vi "Config Spark Max SLOT SmartMotion HW Get Set.vi"(4 "PIDF Slot (0)":i32, 6 "Get(f) Set(t)":bool, 7 "SparkMax Slot SM":T1={"Max Velocity"=0.0, "Max Acceleration"=1.0, "Allowed CL Error"=0.0, "Min Velocity Output"=0.0}, 8 "Error":errorcluster, 11 "Drive Refs":T2) -> (0 "Error Out":errorcluster, 3 "Drive Refs Out":T2, 5 "SparkMax Slot SM Out":T1={"Max Velocity"=0.0, "Max Acceleration"=1.0, "Allowed CL Error"=0.0, "Min Velocity Output"=0.0})   [LabVIEW 2023, in "Swerve AM_ACT.lvlib"]
uses:
  Swerve AM_ACT.lvlib
  <vilib>/Rock Robotics/WPI/MotorControl/WPI_MotorControlDeviceRef.ctl
  <vilib>/Rock Robotics/WPI/MotorControl/WPI_MotorControlType.ctl
  <vilib>/Rock Robotics/SystemInterfaces/DIO/FPGA_DIOPWMChannel.ctl
  <vilib>/Rock Robotics/WPI/PWM/WPI_PWMDeadband.ctl
  <vilib>/Rock Robotics/SystemInterfaces/DIO/FPGA_DIOChannel.ctl
  Shared Code/TypeDefs/Cluster_SparkMax Smart Motion Parameters.ctl
  Shared Code/TypeDefs/Cluster_SRX SLOT PID Config.ctl
  Shared Code/TypeDefs/Cluster_PID Gains.ctl
  <vilib>/Utility/error.llb/Trim Whitespace One-Sided.vi
  <vilib>/Utility/Data Type/NI_Data Type.lvlib
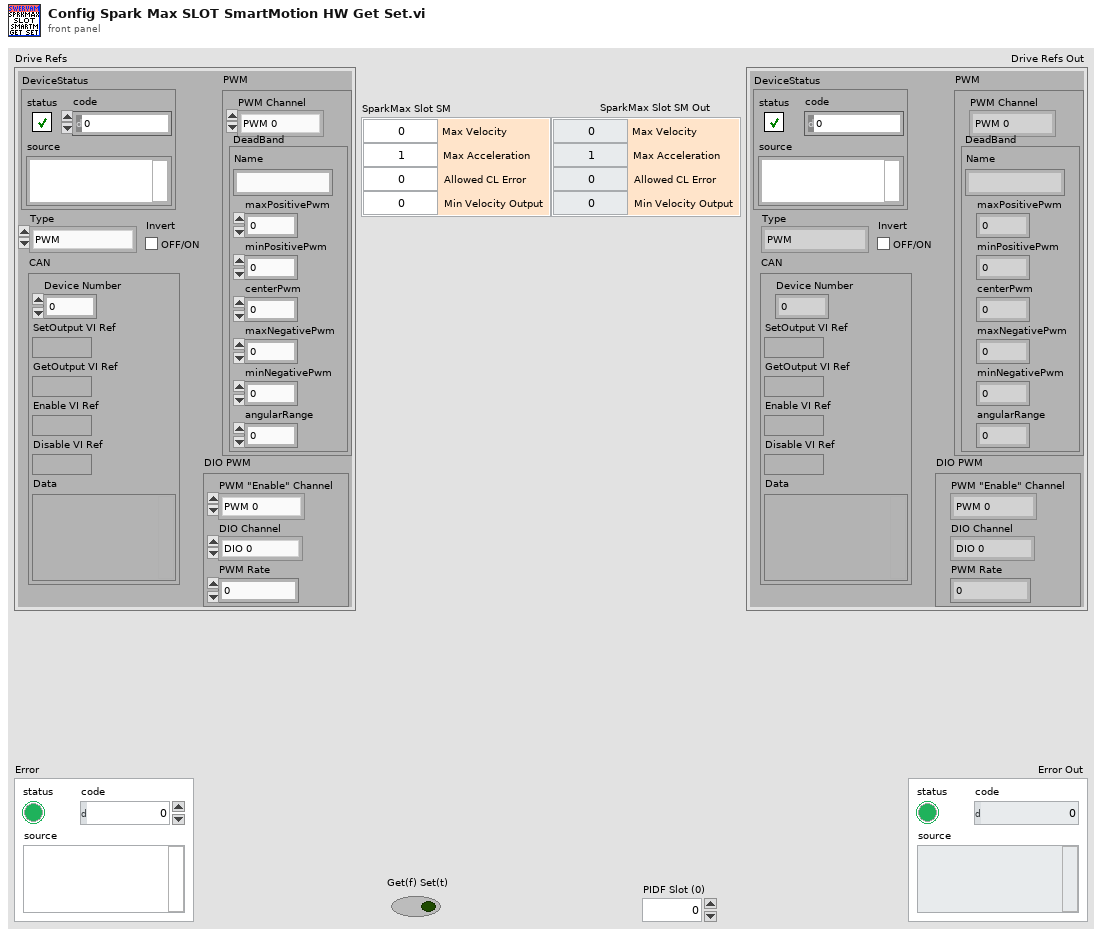
[diagram p1: front panel]
types:
  T1 = typedef "Cluster_SparkMax Smart Motion Parameters.ctl" = cluster{"Max Velocity":dbl, "Max Acceleration":dbl, "Allowed CL Error":dbl, "Min Velocity Output":dbl}
  T2 = typedef "WPI_MotorControlDeviceRef.ctl" = cluster{"DeviceStatus":errorcluster, "Type":T3, "PWM":cluster{"PWM Channel":T4, "DeadBand":T5}, "CAN":cluster{"Device Number":u8, "SetOutput VI Ref":variant, "GetOutput VI Ref":variant, "Enable VI Ref":variant, "Disable VI Ref":variant, "Data":variant}, "Invert":bool, "DIO PWM":cluster{"PWM \"Enable\" Channel":T4, "DIOChannel":T6, "PWM Rate":dbl}}
  T3 = typedef "WPI_MotorControlType.ctl" = enum16{"PWM", "CAN", "DIO PWM"}
  T4 = typedef "FPGA_DIOPWMChannel.ctl" = enum8{"PWM 0", "PWM 1", "PWM 2", "PWM 3", "PWM 4", "PWM 5", "PWM 6", "PWM 7", "PWM 8", "PWM 9", "PWM MXP 0", "PWM MXP 1", "PWM MXP 2", "PWM MXP 3", "PWM MXP 4", "PWM MXP 5", "PWM MXP 6", "PWM MXP 7", "PWM MXP 8", "PWM MXP 9", "Invalid"}
  T5 = typedef "WPI_PWMDeadband.ctl" = cluster{"Name":string, "maxPositivePwm":i32, "minPositivePwm":i32, "centerPwm":i32, "maxNegativePwm":i32, "minNegativePwm":i32, "angularRange":u16}
  T6 = typedef "FPGA_DIOChannel.ctl" = enum8{"DIO 0", "DIO 1", "DIO 2", "DIO 3", "DIO 4", "DIO 5", "DIO 6", "DIO 7", "DIO 8", "DIO 9", "DIO MXP 0", "DIO MXP 1", "DIO MXP 2", "DIO MXP 3", "DIO MXP 4", "DIO MXP 5", "DIO MXP 6", "DIO MXP 7", "DIO MXP 8", "DIO MXP 9", "DIO MXP 10", "DIO MXP 11", "DIO MXP 12", "DIO MXP 13", "DIO MXP 14", "DIO MXP 15", "SPI Port CS1", "SPI Port CS2", "SPI Port CS3", "SPI Port MISO", "SPI Port MOSI", "Invalid"}
  T7 = typedef "Cluster_SRX SLOT PID Config.ctl" = cluster{"Gains":T8, "Error Allowed":dbl, "I Zone":dbl, "Peak Out 0-1":dbl, "Max I Accu":dbl}
  T8 = typedef "Cluster_PID Gains.ctl" = cluster{"P":dbl, "I":dbl, "D":dbl, "F":dbl}
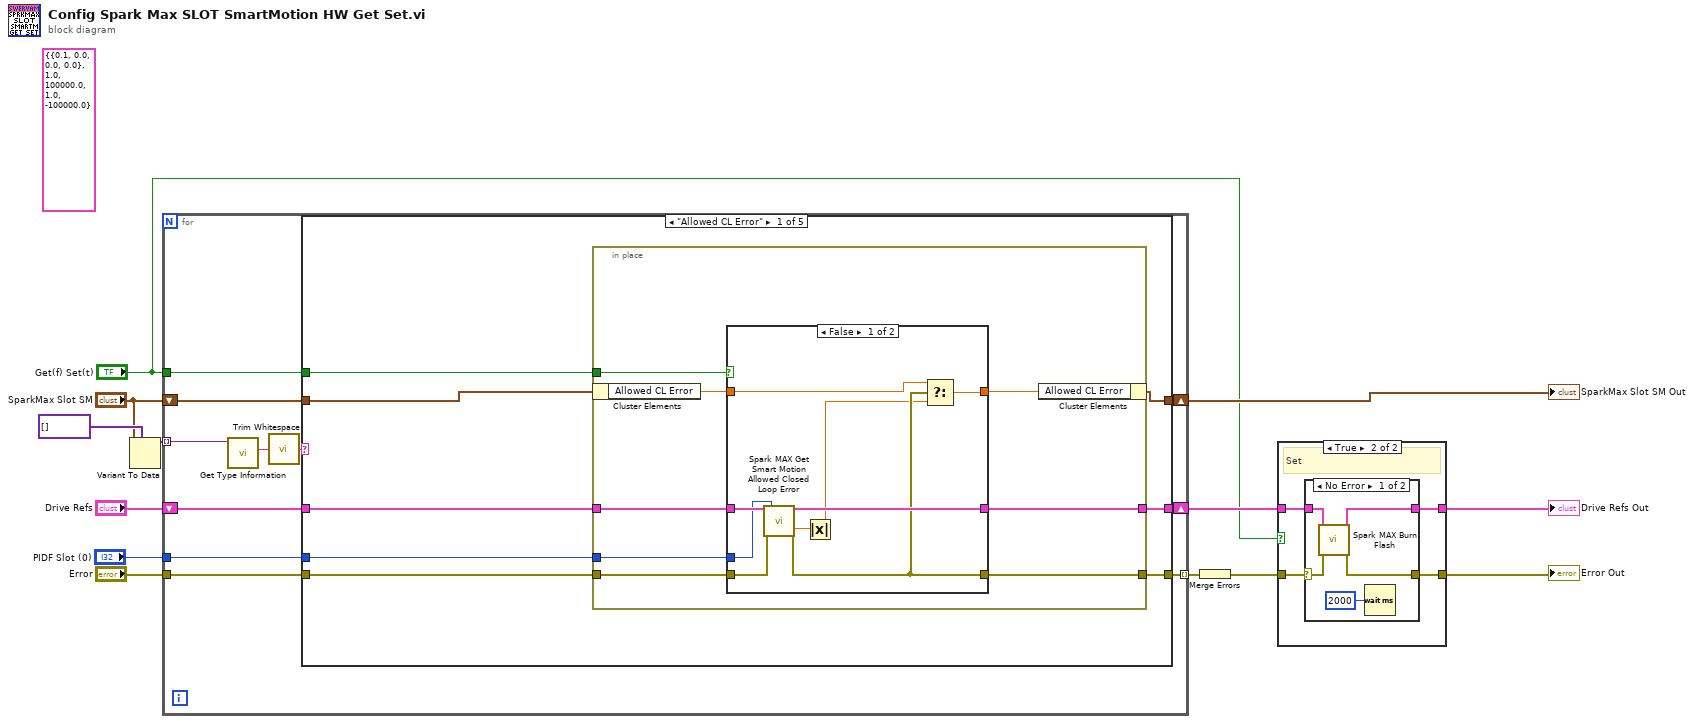
[diagram p0: block diagram]
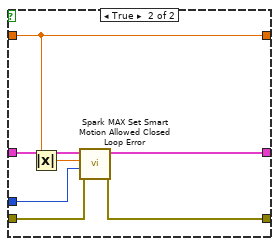
[diagram p4: hidden frame]
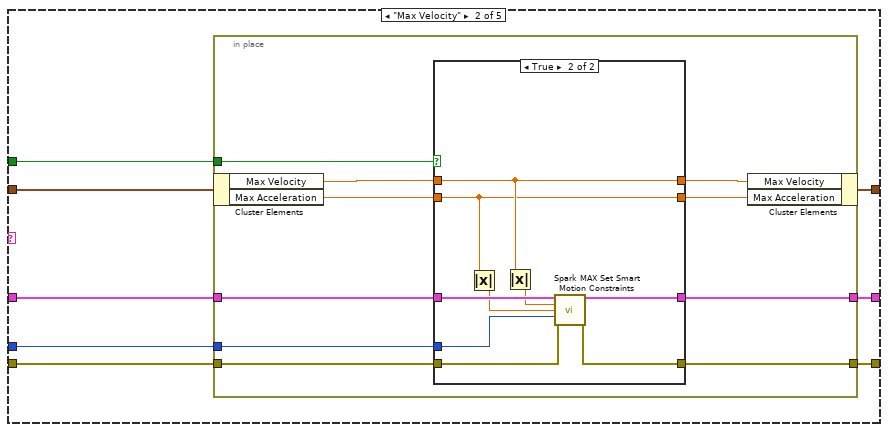
[diagram p5: hidden frame]
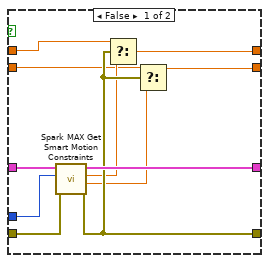
[diagram p6: hidden frame]
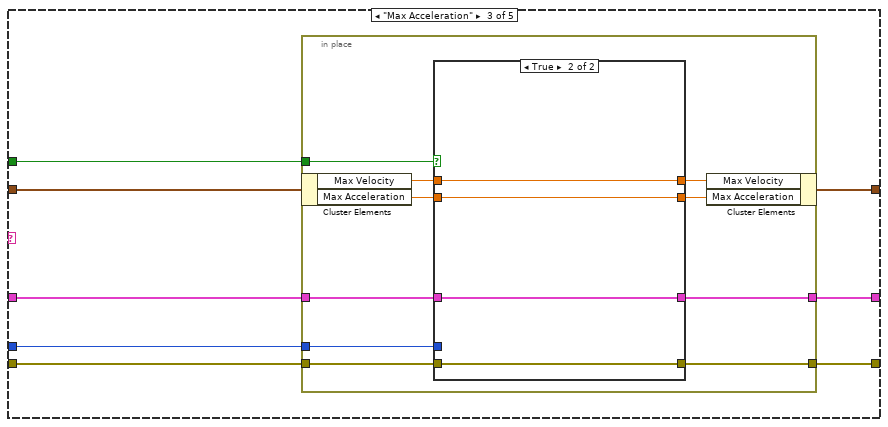
[diagram p7: hidden frame]
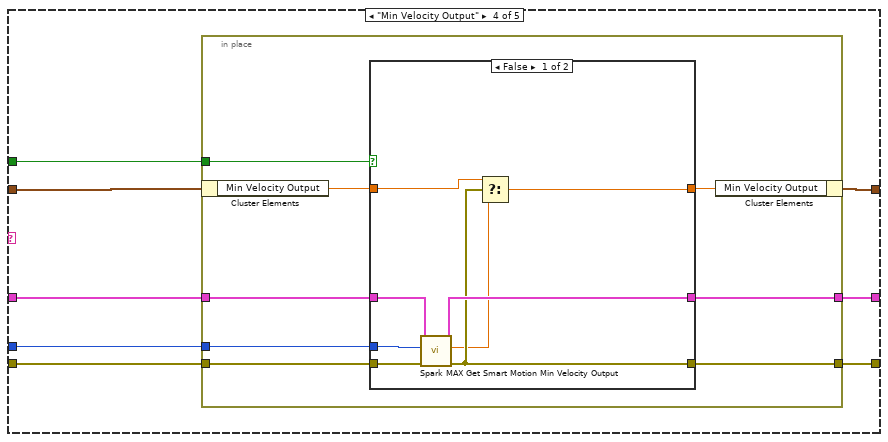
[diagram p9: hidden frame]
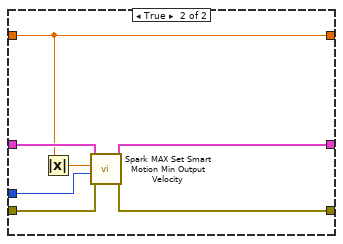
[diagram p10: hidden frame]
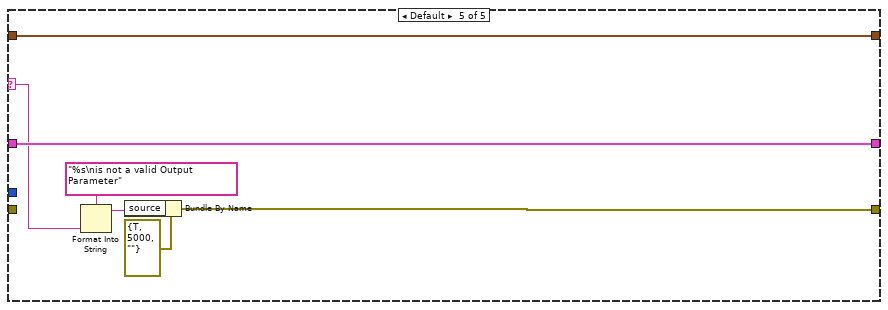
[diagram p11: hidden frame]
diagram:
  (unwired) T7 {"Gains"={"P"=0.1, "I"=0.0, "D"=0.0, "F"=0.0}, "Error Allowed"=1.0, "I Zone"=100000.0, "Peak Out 0-1"=1.0, "Max I Accu"=-100000.0} ("SparkMax Output")
  n1 = Variant To Data(type=variant[] [], Variant="SparkMax Slot SM") -> (data=w10:variant[])  [unwired: 1 in, 1 out]
  n2 = for {
    shift-right: [w15] -> w13
    shift-left: "SparkMax Slot SM" -> [w21]
    shift-right: [w16] -> w3
    shift-left: "Drive Refs" -> [w20]
    tunnel: "Get(f) Set(t)" -> [w19]
    tunnel: w10 -> [w23] mode=indexing
    tunnel: "Error" -> [w18]
    tunnel: [w17] -> w7 mode=indexing
    tunnel: "PIDF Slot (0)" -> [w14]
    n3 = call <vilib>:"Get Type Information.vi"("variant"=w23) -> ("name"=w24:string)  [unwired: 6 in, 4 out]
    n4 = call <vilib>:"Trim Whitespace.vi"("string"=w24) -> ("trimmed string"=w22:string)  [unwired: 1 in]
    n5 = case shown="\"Allowed CL Error\"" w22 {
      selector: w22 -> [_ _ _ _ w156]
      tunnel: w21 -> [w32 w64 w102 w128 w158]
      tunnel: w20 -> [w28 w60 w98 w124 w157]
      tunnel: w19 -> [w31 w63 w101 w127 _]
      tunnel: w18 -> [w30 w62 w100 w126 _]
      tunnel: [w29 w61 w99 w125 w154] -> w17
      tunnel: [w27 w59 w97 w123 w157] -> w16
      tunnel: [w26 w58 w96 w122 w158] -> w15
      tunnel: w14 -> [w25 w57 w95 w121 _]
      frame "Allowed CL Error" {
        n6 = in-place {
          in-place-border: w31 -> [w40]
          in-place-border: w30 -> [w38]
          in-place-border: [w37] -> w29
          in-place-border: w28 -> [w36]
          in-place-border: [w35] -> w27
          in-place-border: w25 -> [w33]
          n7 = in-place-cluster #1(w32) -> ("Allowed CL Error"=w39:dbl)
          n8 = case shown="False" w40 {
            tunnel: w39 -> [w43 w56]
            tunnel: w38 -> [w45 w53]
            tunnel: [w44 w52] -> w37
            tunnel: w36 -> [w47 w55]
            tunnel: [w48 w54] -> w35
            tunnel: [w49 w56] -> w34
            tunnel: w33 -> [w46 w51]
            frame False {
              n9 = call <vilib>:"Spark MAX Get Smart Motion Allowed Closed Loop Error.vi"("MotorControlDeviceRef"=w47, "error in"=w45, "PIDF Slot (0)"=w46) -> ("MotorControlDeviceRef"=w48:T2, "Allowed Closed Loop Error"=w42:dbl, "error out"=w44:errorcluster)  [unwired: 14 in]
              n10 = Absolute Value(x=w42) -> (abs(x)=w41:dbl)
              n11 = Select(t=w43, s=w44, f=w41) -> (s? t:f=w49:dbl)
            }
            frame True {
              n12 = Absolute Value(x=w56) -> (abs(x)=w50:dbl)
              n13 = call <vilib>:"Spark MAX Set Smart Motion Allowed Closed Loop Error.vi"("error in"=w53, "PIDF Slot (0)"=w51, "Allowed Closed Loop Error"=w50, "MotorControlDeviceRef"=w55) -> ("error out"=w52:errorcluster, "MotorControlDeviceRef"=w54:T2)  [unwired: 6 in]
            }
          }
          n14 = in-place-cluster #1("Allowed CL Error"=w34) -> (w26:T1)
        }
      }
      frame "Max Velocity" {
        n15 = in-place {
          in-place-border: w63 -> [w74]
          in-place-border: w62 -> [w72]
          in-place-border: [w71] -> w61
          in-place-border: w60 -> [w70]
          in-place-border: [w69] -> w59
          in-place-border: w57 -> [w67]
          n16 = in-place-cluster #2(w64) -> ("Max Velocity"=w73:dbl, "Max Acceleration"=w66:dbl)
          n17 = case shown="True" w74 {
            tunnel: w73 -> [w76 w94]
            tunnel: w72 -> [w83 w91]
            tunnel: [w81 w90] -> w71
            tunnel: w70 -> [w85 w93]
            tunnel: [w84 w92] -> w69
            tunnel: [w77 w94] -> w68
            tunnel: w67 -> [w82 w87]
            tunnel: w66 -> [w75 w86]
            tunnel: [w79 w86] -> w65
            frame False {
              n18 = call <vilib>:"Spark MAX Get Smart Motion Constraints.vi"("error in"=w83, "PIDF Slot (0)"=w82, "MotorControlDeviceRef"=w85) -> ("error out"=w81:errorcluster, "Max Acceleration"=w80:dbl, "Max Velocity"=w78:dbl, "MotorControlDeviceRef"=w84:T2)  [unwired: 5 in]
              n19 = Select(t=w76, s=w81, f=w78) -> (s? t:f=w77:dbl)
              n20 = Select(t=w75, s=w81, f=w80) -> (s? t:f=w79:dbl)
            }
            frame True {
              n21 = Absolute Value(x=w86) -> (abs(x)=w88:dbl)
              n22 = Absolute Value(x=w94) -> (abs(x)=w89:dbl)
              n23 = call <vilib>:"Spark MAX Set Smart Motion Constraints.vi"("MotorControlDeviceRef"=w93, "Max Velocity"=w89, "Max Acceleration"=w88, "PIDF Slot (0)"=w87, "error in"=w91) -> ("MotorControlDeviceRef"=w92:T2, "error out"=w90:errorcluster)  [unwired: 9 in]
            }
          }
          n24 = in-place-cluster #2("Max Velocity"=w68, "Max Acceleration"=w65) -> (w58:T1)
        }
      }
      frame "Max Acceleration" {
        n25 = in-place {
          in-place-border: w101 -> [w112]
          in-place-border: w100 -> [w110]
          in-place-border: [w109] -> w99
          in-place-border: w98 -> [w108]
          in-place-border: [w107] -> w97
          in-place-border: w95 -> [w105]
          n26 = in-place-cluster #3(w102) -> ("Max Velocity"=w111:dbl, "Max Acceleration"=w104:dbl)
          n27 = case shown="True" w112 {
            tunnel: w111 -> [w116 w120]
            tunnel: w110 -> [w114 w117]
            tunnel: [w114 w117] -> w109
            tunnel: w108 -> [w113 w118]
            tunnel: [w113 w118] -> w107
            tunnel: [w116 w120] -> w106
            tunnel: w105 -> [_ _]
            tunnel: w104 -> [w115 w119]
            tunnel: [w115 w119] -> w103
            frame False {
            }
            frame True {
            }
          }
          n28 = in-place-cluster #3("Max Velocity"=w106, "Max Acceleration"=w103) -> (w96:T1)
        }
      }
      frame "Min Velocity Output" {
        n29 = in-place {
          in-place-border: w127 -> [w136]
          in-place-border: w126 -> [w134]
          in-place-border: [w133] -> w125
          in-place-border: w124 -> [w132]
          in-place-border: [w131] -> w123
          in-place-border: w121 -> [w129]
          n30 = in-place-cluster #4(w128) -> ("Min Velocity Output"=w135:dbl)
          n31 = case shown="False" w136 {
            tunnel: w135 -> [w143 w145]
            tunnel: w134 -> [w140 w151]
            tunnel: [w139 w150] -> w133
            tunnel: w132 -> [w142 w148]
            tunnel: [w141 w147] -> w131
            tunnel: [w144 w145] -> w130
            tunnel: w129 -> [w138 w149]
            frame False {
              n32 = call <vilib>:"Spark MAX Get Smart Motion Min Velocity Output.vi"("error in"=w140, "PIDF Slot (0)"=w138, "MotorControlDeviceRef"=w142) -> ("error out"=w139:errorcluster, "Minimum Velocity Output"=w137:dbl, "MotorControlDeviceRef"=w141:T2)  [unwired: 6 in]
              n33 = Select(t=w143, s=w139, f=w137) -> (s? t:f=w144:dbl)
            }
            frame True {
              n34 = Absolute Value(x=w145) -> (abs(x)=w146:dbl)
              n35 = call <vilib>:"Spark MAX Set Smart Motion Min Output Velocity.vi"("error in"=w151, "PIDF Slot (0)"=w149, "Minimum Velocity Output"=w146, "MotorControlDeviceRef"=w148) -> ("error out"=w150:errorcluster, "MotorControlDeviceRef"=w147:T2)  [unwired: 6 in]
            }
          }
          n36 = in-place-cluster #4("Min Velocity Output"=w130) -> (w122:T1)
        }
      }
      frame Default {
        n37 = Format Into String(format string="%s\nis not a valid Output Parameter", w156) -> (resulting string=w152:string)  [unwired: 2 in, 1 out]
        n38 = Bundle By Name(cluster=errorcluster {"status"=TRUE, "code"=5000, "source"=""} ("error out"), "source"=w152) -> (w154:errorcluster)
      }
    }
  }
  "SparkMax Slot SM Out" <- w13
  n39 = Merge Errors(w7) -> (w5:errorcluster)
  n40 = case shown="True" "Get(f) Set(t)" {
    tunnel: w5 -> [w159 w164]
    tunnel: [w159 w163] -> w4
    tunnel: w3 -> [w160 w162]
    tunnel: [w160 w161] -> w2
    frame False {
      # "Get"
    }
    frame True {
      # "Set"
      n41 = case shown="No Error" w164 {
        selector: w164 -> [w169 w170]
        tunnel: [w168 w170] -> w163
        tunnel: w162 -> [w167 w171]
        tunnel: [w166 w171] -> w161
        frame No Error {
          n42 = call <vilib>:"Spark MAX Burn Flash.vi"("error in"=w169, "MotorControlDeviceRef"=w167) -> ("error out"=w168:errorcluster, "MotorControlDeviceRef"=w166:T2)  [unwired: 8 in]
          n43 = Wait (ms)(milliseconds to wait=u32 2000) -> ()  [unwired: 1 out]
        }
        frame Error {
        }
      }
    }
  }
  "Error Out" <- w4
  "Drive Refs Out" <- w2
